vi "Read dRA_sps.vi"(8 "error in (no error)":errorcluster, 11 "DifftrackRADec in":refnum<class "DifftrackRADec.lvclass">) -> (0 "error out":errorcluster, 2 "dRA_sps":dbl min=0.0 max=10.0, 3 "DifftrackRADec out":refnum<class "DifftrackRADec.lvclass">)   [LabVIEW 2022 SP3, in "TCSDataDefinitions.lvlib" / "TCSCommand.lvlib" / "TargetConfiguration.lvlib" / "Target.lvlib" / "DifftrackRADec.lvclass"]
uses:
  DifftrackRADec.lvclass
  DifftrackRADec.lvclass/DifftrackRADec.ctl
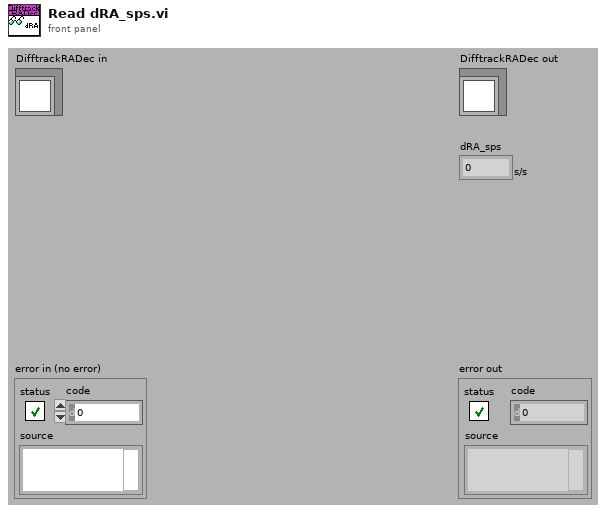
[diagram p1: front panel]
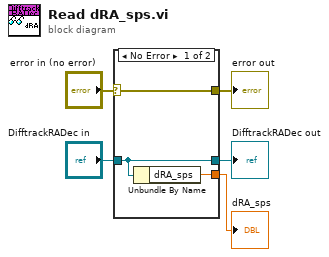
[diagram p0: block diagram]
diagram:
  n1 = case shown="No Error" "error in (no error)" {
    selector: "error in (no error)" -> [w8 w9]
    tunnel: [w8 w9] -> w4
    tunnel: [w7 w10] -> w2
    tunnel: "DifftrackRADec in" -> [w7 w10]
    tunnel: [w6 _] -> w1
    frame No Error {
      n2 = Unbundle By Name(w7) -> ("dRA_sps"=w6:dbl)
    }
    frame Error {
    }
  }
  "error out" <- w4
  "DifftrackRADec out" <- w2
  "dRA_sps" <- w1
